vi "Actor Core.vi"(8 "error in":errorcluster, 11 "Sample Line in":refnum<class "Sample Line.lvclass">) -> (0 "error out":errorcluster, 3 "Actor out":refnum<class "Actor.lvclass">)   [LabVIEW 2015, in "cRIO-Carbondioxide.lvlib" / "CO2-Actor.lvlib" / "Sample Line.lvclass"]
doc: "(<B>Filename</B>: Actor Framework.lvlib:Actor.lvclass:Actor Core.vi)\n\nReceives messages to the actor, reacts to them, and initiates any error handling that may shut the actor down.\n\nDescendant classes may override this VI to append parallel tasks for the actor to complete while it handles messages. Overrides use the Call Parent Method node."
uses:
  Sample Line.lvclass
  <vilib>/ActorFramework/Actor/Actor.lvclass
  Sample Line.lvclass/Sample Line.ctl
  CO2 Actor/CO2 Actor.lvclass
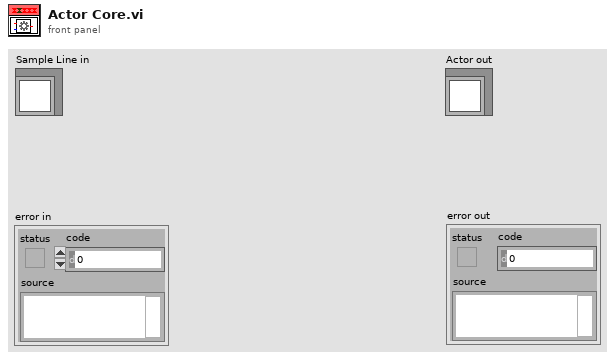
[diagram p1: front panel]
types:
  T1 = typedef "Sample Container.ctl" = cluster{"Sample In":refnum<k21>, "Sample Name":refnum<k21>, "Ti Cathode":refnum<k21>, "SampleQ":refnum<queue>}
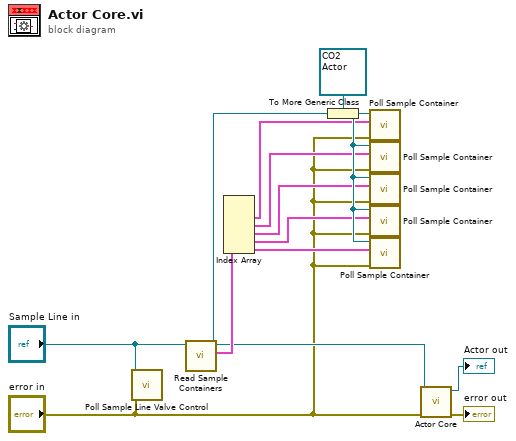
[diagram p0: block diagram]
diagram:
  n1 = call "Poll Sample Line Valve Control.vi"("error in (no error)"="error in", "Sample Line in"="Sample Line in") -> ()  [unwired: 10 in]
  n2 = call "Read Sample Containers.vi"("Sample Line in"="Sample Line in") -> ("Sample Containers"=w4:T1[], "Sample Line out"=w2:refnum<class "Sample Line.lvclass">)  [unwired: 9 in]
  n3 = Index Array(array=w4) -> (element #1=w9:T1, element #2=w8:T1, element #3=w7:T1, element #4=w6:T1, element #5=w5:T1)  [unwired: 5 in]
  n4 = To More Generic Class(target class=refnum<class "CO2 Actor.lvclass"> refnum ("CO2 Actor in"), reference=w2) -> (generic class reference=w10:refnum<class "CO2 Actor.lvclass">)
  n5 = call-dynamic "Poll Sample Container.vi"("error in (no error)"="error in", "Sample Container"=w9, "CO2 Actor in"=w10) -> ()  [unwired: 8 in, 1 out]
  n6 = call-dynamic "Poll Sample Container.vi"("error in (no error)"="error in", "Sample Container"=w8, "CO2 Actor in"=w10) -> ()  [unwired: 8 in, 1 out]
  n7 = call-dynamic "Poll Sample Container.vi"("error in (no error)"="error in", "Sample Container"=w7, "CO2 Actor in"=w10) -> ()  [unwired: 8 in, 1 out]
  n8 = call-dynamic "Poll Sample Container.vi"("error in (no error)"="error in", "Sample Container"=w6, "CO2 Actor in"=w10) -> ()  [unwired: 8 in, 1 out]
  n9 = call-dynamic "Poll Sample Container.vi"("error in (no error)"="error in", "Sample Container"=w5, "CO2 Actor in"=w10) -> ()  [unwired: 8 in, 1 out]
  n10 = call-parent "Actor Core.vi"("error in"="error in", "CO2 Actor in"=w2) -> ("error out"=→"error out":errorcluster, "Actor out"=→"Actor out":refnum<class "Actor.lvclass">)  [unwired: 8 in]
